vi "test_Format Numeric To String_double to string using Format Value node (No format string).vi"(8 "error in (no error)":errorcluster, 11 "TestCase in":refnum<class "Instrument Addon Unit Tests.lvclass">) -> (0 "error out":errorcluster, 3 "TestCase out":refnum<class "Instrument Addon Unit Tests.lvclass">)   [LabVIEW 2020, in "Instrument Addon Unit Tests.lvclass"]
uses:
  Instrument Addon Unit Tests.lvclass
  Addon/Addon Shared/Types/Metadata Channel Type.ctl
  <vilib>/addons/_JKI Toolkits/VI Tester/TestCase.llb/TestCase.lvclass
  Addon/Addon Engine/Instrument Addon Engine.lvlib
  Addon/Addon Shared/Instrument Addon Shared.lvlib
  C:/Program Files (x86)/National Instruments/LabVIEW 2020/vi.lib/addons/_JKI Toolkits/VI Tester/TestCase.llb/TestCase.lvclass
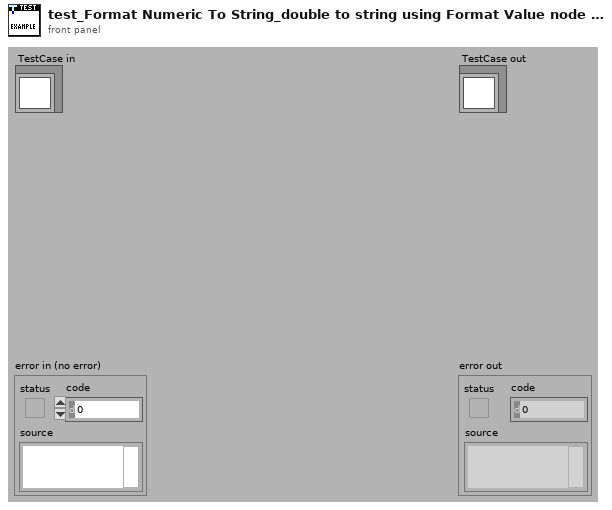
[diagram p1: front panel]
types:
  T1 = typedef "Instrument Addon Shared.lvlib/Metadata Channel Type.ctl" = enum16{"Enumerated List", "Format", "Type Cast"}
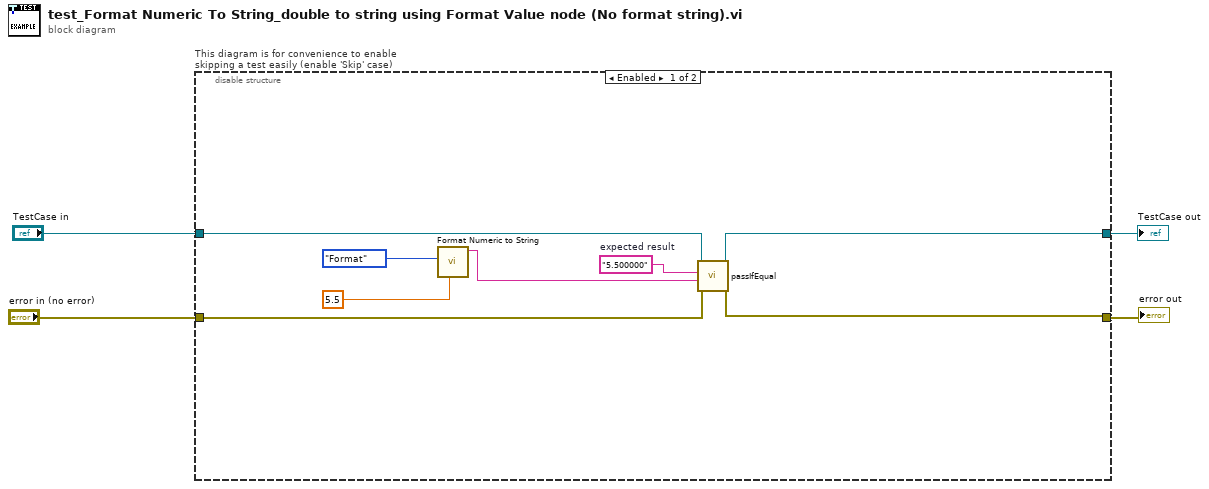
[diagram p0: block diagram]
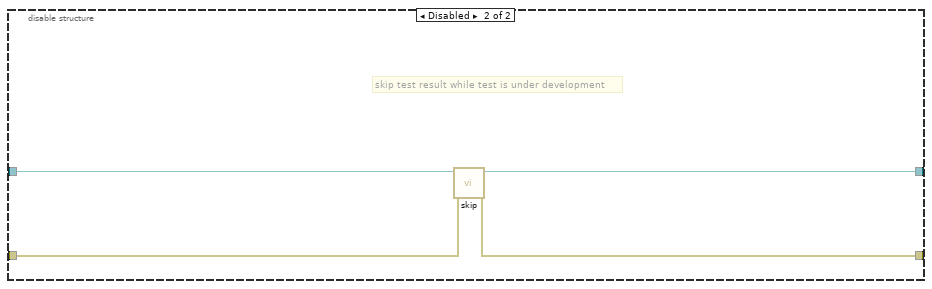
[diagram p2: hidden frame]
diagram:
  n1 = disable-structure "This diagram is for convenience to enable skipping a test easily (enable 'Skip' case)" shown="Enabled" {
    disable-tunnel: "TestCase in" -> [w11 w16]
    disable-tunnel: [w10 w14] -> w1
    disable-tunnel: [w9 w15] -> w3
    disable-tunnel: "error in (no error)" -> [w6 w13]
    frame Enabled {
      w12 = "5.500000"  # expected result
      n2 = call "Format Numeric to String.vi"("Numeric"=5.5, "Channel Type"=Metadata_Channel_Type."Format") -> ("Value"=w7:string)  [unwired: 9 in]
      n3 = call-dynamic "passIfEqual.vi"("error in (no error)"=w6, "y"=w7, "x"=w12, "TestCase in"=w11) -> ("error out"=w9:errorcluster, "TestCase out"=w10:refnum<class "Instrument Addon Unit Tests.lvclass">)  [unwired: 6 in]
    }
    frame Disabled {
      # "skip test result while test is under development"
      n4 = call <vilib>:"skip.vi"("error in (no error)"=w13, "TestCase in"=w16) -> ("error out"=w15:errorcluster, "TestCase out"=w14:refnum<class "Instrument Addon Unit Tests.lvclass">)  [unwired: 8 in]
    }
  }
  "error out" <- w3
  "TestCase out" <- w1
